vi "Initialize.vi"(8 "error in (no error)":errorcluster, 9 "Reset (True)":bool=TRUE, 10 "ID Query (True)":bool=TRUE, 11 "VISA resource name":refnum<visa-resource-name>) -> (0 "error out":errorcluster, 3 "VISA resource name out":refnum<visa-resource-name>)   [LabVIEW 2015, in "BK Precision 983X Series.lvlib"]
doc: "Establishes communication with the instrument and optionally performs an instrument identification query and/or an instrument reset. It also places the instrument in a default state needed for other instrument driver operations. Therefore, call this VI before calling other instrument driver VIs for this instrument. Generally, you need to call the Initialize VI only once at the beginning of an application."
uses:
  <instrlib>/BK Precision 983X Series/BK Precision 983X Series.lvlib
panel:
  # "(c) 2017 B&K Precision Corporation.  ALL RIGHTS RESERVED."
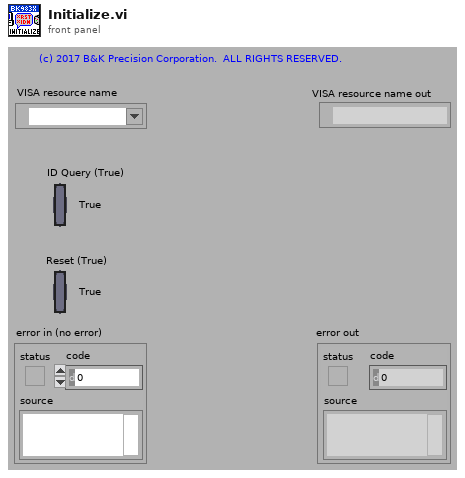
[diagram p1: front panel]
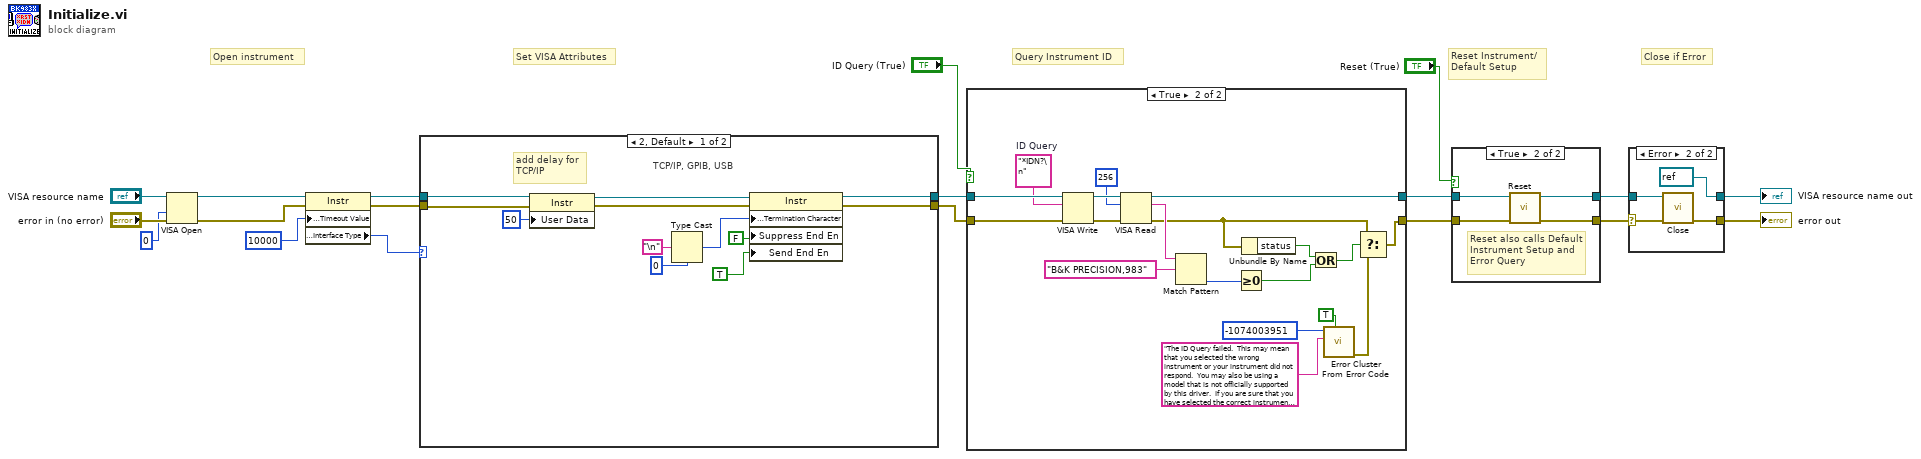
[diagram p0: block diagram]
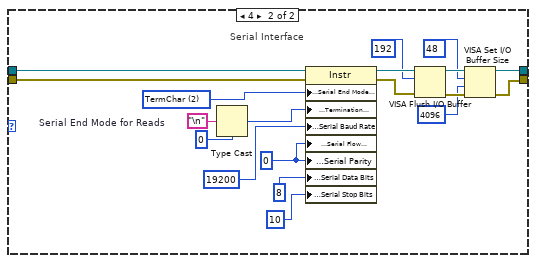
[diagram p2: hidden frame]
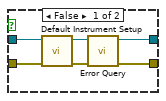
[diagram p4: hidden frame]
diagram:
  # "Set VISA Attributes"
  # "Close if Error"
  # "Query Instrument ID"
  # "Reset Instrument/\nDefault Setup"
  # "Open instrument"
  n1 = VISA Open(access mode=u32 0, error in (no error)="error in (no error)", VISA resource name="VISA resource name") -> (VISA resource name=w3:refnum<visa-resource-name>, error out=w2:errorcluster)  [unwired: 2 in]
  n2 = property class="Instr"(reference=w3, error in=w2, "General Settings:Timeout Value"=u32 10000) -> (reference out=w10:refnum<visa-resource-name>, error out=w9:errorcluster, "Interface Information:Interface Type"=w1:u16)
  n3 = case shown="2, Default" w1 {
    tunnel: [w25 w47] -> w12
    tunnel: [w26 w44] -> w11
    tunnel: w10 -> [w24 w49]
    tunnel: w9 -> [w23 w50]
    frame 2, Default {
      # "add delay for\nTCP/IP"
      # "TCP/IP, GPIB, USB"
      n4 = property class="Instr"(reference=w24, error in=w23, "User Data"=u32 50 ("General Settings:User Data")) -> (reference out=w22:refnum<visa-resource-name>, error out=w21:errorcluster)
      n5 = Type Cast(type=u8 0, x="\n" ("Line Feed Constant")) -> (*(type *) &x=w29:u8)
      n6 = property class="Instr"(reference=w22, error in=w21, "Message Based Settings:Termination Character"=w29, "Suppress End En"=FALSE, "Send End En"=TRUE) -> (reference out=w25:refnum<visa-resource-name>, error out=w26:errorcluster)
    }
    frame 4 {
      w34 = 0
      w37 = u16 2 items=["None", "LastBit", "TermChar"]  # Serial End Mode for Reads
      # "Serial Interface"
      n7 = Type Cast(type=u8 0, x="\n" ("Line Feed Constant")) -> (*(type *) &x=w36:u8)
      n8 = property class="Instr"(reference=w49, error in=w50, "Serial Settings:Serial End Mode for Reads"=w37, "Message Based Settings:Termination Character"=w36, "Serial Settings:Serial Baud Rate"=19200, "Serial Settings:Serial Flow Control"=w34, "Serial Settings:Serial Parity"=w34, "Serial Settings:Serial Data Bits"=8, "Serial Settings:Serial Stop Bits"=10) -> (reference out=w43:refnum<visa-resource-name>, error out=w46:errorcluster)
      n9 = VISA Flush I/O Buffer(VISA resource name=w43, mask (16)=u16 192, error in (no error)=w46) -> (VISA resource name out=w48:refnum<visa-resource-name>, error out=w45:errorcluster)
      n10 = VISA Set I/O Buffer Size(VISA resource name=w48, mask (16)=u16 48, size (4096)=u32 4096 ("size (0)"), error in (no error)=w45) -> (VISA resource name out=w47:refnum<visa-resource-name>, error out=w44:errorcluster)
    }
  }
  n11 = case shown="True" "ID Query (True)" {
    tunnel: [w51 w71] -> w18
    tunnel: [w52 w68] -> w19
    tunnel: w12 -> [w52 w69]
    tunnel: w11 -> [w51 w70]
    frame False {
    }
    frame True {
      w62 = "*IDN?\n"  # ID Query
      n12 = VISA Write(VISA resource name=w69, write buffer=w62, error in (no error)=w70) -> (VISA resource name out=w66:refnum<visa-resource-name>, error out=w65:errorcluster)  [unwired: 1 out]
      n13 = VISA Read(VISA resource name=w66, byte count=u32 256, error in (no error)=w65) -> (VISA resource name out=w68:refnum<visa-resource-name>, read buffer=w67:string, error out=w56:errorcluster)  [unwired: 1 out]
      n14 = Match Pattern(string=w67, regular expression="B&K PRECISION,983") -> (offset past match=w57:i32)  [unwired: 1 in, 3 out]
      n15 = Greater Or Equal To 0?(x=w57) -> (x >= 0?=w54:bool)
      n16 = Unbundle By Name(w56) -> ("status"=w55:bool)
      n17 = Or(x=w55, y=w54) -> (x .or. y?=w53:bool)
      n18 = call <vilib>:"Error Cluster From Error Code.vi"("show call chain? (False)"=TRUE, "error message (\"\")"="The ID Query failed.  This may mean that you selected the wrong instrument or your instrument did not respond.  You may also be using a model that is not officially supported by this driver.  If you are sure that you have selected the correct instrument and it is responding, try disabling the ID Query." ("Source (VI Name)"), "error code (0)"=-1074003951 ("Code")) -> ("error out"=w61:errorcluster)  [unwired: 6 in]
      n19 = Select(t=w56, s=w53, f=w61) -> (s? t:f=w71:errorcluster)
    }
  }
  n20 = case shown="True" "Reset (True)" {
    tunnel: w18 -> [w76 w78]
    tunnel: [w73 w81] -> w4
    tunnel: w19 -> [w77 w79]
    tunnel: [w74 w80] -> w5
    frame False {
      n21 = call <instrlib>:"Default Instrument Setup.vi"("error in (no error)"=w76, "VISA resource name"=w77) -> ("error out"=w72:errorcluster, "VISA resource name out"=w75:refnum<visa-resource-name>)  [unwired: 8 in]
      n22 = call <instrlib>:"Error Query.vi"("error in (no error)"=w72, "VISA resource name"=w75) -> ("error out"=w73:errorcluster, "VISA resource name out"=w74:refnum<visa-resource-name>)  [unwired: 6 in, 2 out]
    }
    frame True {
      # "Reset also calls Default Instrument Setup and Error Query"
      n23 = call <instrlib>:"Reset.vi"("error in (no error)"=w78, "VISA resource name"=w79) -> ("error out"=w81:errorcluster, "VISA resource name out"=w80:refnum<visa-resource-name>)  [unwired: 8 in]
    }
  }
  n24 = case shown="Error" w4 {
    selector: w4 -> [w82 w85]
    tunnel: w5 -> [w83 w86]
    tunnel: [w83 refnum<visa-resource-name> refnum ("VISA resource name out")] -> w7
    tunnel: [w82 w87] -> w6
    frame No Error {
    }
    frame Error {
      n25 = call <instrlib>:"Close.vi"("error in (no error)"=w85, "VISA resource name"=w86) -> ("error out"=w87:errorcluster)  [unwired: 9 in]
    }
  }
  "VISA resource name out" <- w7
  "error out" <- w6
